vi "Wait Lockin Start.vi"(8 "error in (no error)":errorcluster, 11 "MeasurementSMO in":refnum<class "MeasurementSMO.lvclass">) -> (0 "error out":errorcluster, 3 "MeasurementSMO out":refnum<class "MeasurementSMO.lvclass">)   [LabVIEW 2019, in "MeasurementSMO.lvclass"]
uses:
  MeasurementSMO.lvclass
  14575ef7-ffd8-4de4-94d8-a49df30f0b8f.vi
  <userlib>/LevyLab/Lockin-Multichannel/Instrument.Lockin/Instrument.Lockin.lvclass
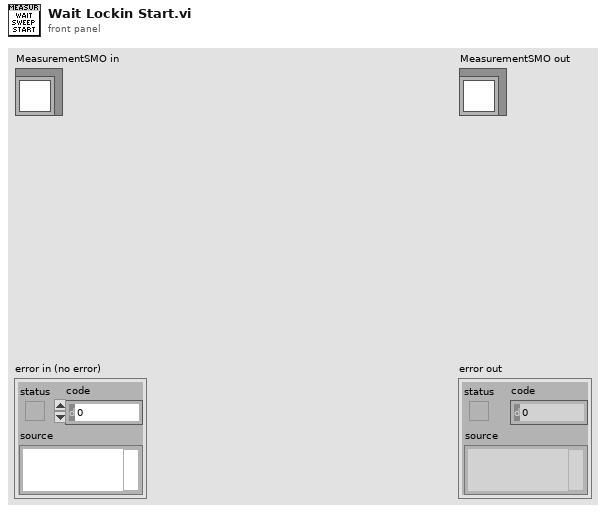
[diagram p1: front panel]
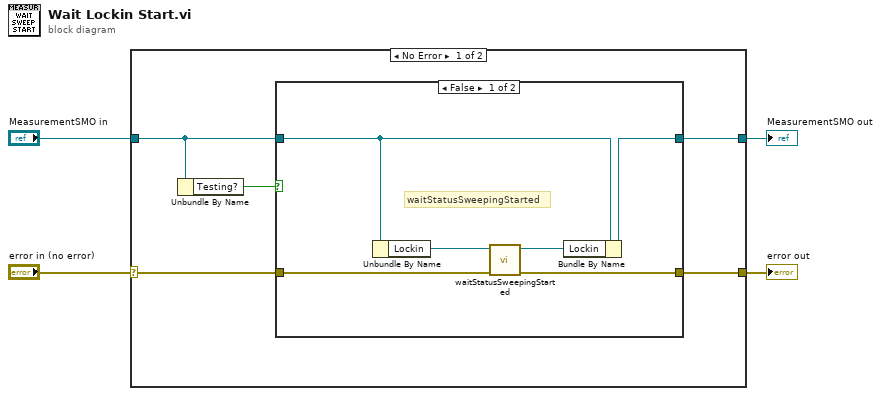
[diagram p0: block diagram]
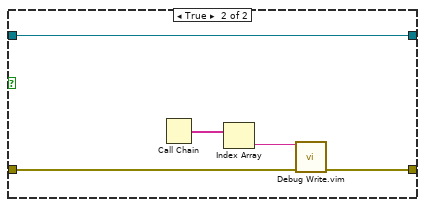
[diagram p2: hidden frame]
diagram:
  n1 = case shown="No Error" "error in (no error)" {
    selector: "error in (no error)" -> [w6 w22]
    tunnel: [w7 w22] -> w3
    tunnel: [w8 w21] -> w1
    tunnel: "MeasurementSMO in" -> [w9 w21]
    frame No Error {
      n2 = Unbundle By Name(w9) -> ("Testing?"=w5:bool)
      n3 = case shown="False" w5 {
        tunnel: w9 -> [w14 w20]
        tunnel: [w15 w20] -> w8
        tunnel: [w10 w19] -> w7
        tunnel: w6 -> [w11 w18]
        frame False {
          # "waitStatusSweepingStarted"
          n4 = Unbundle By Name(w14) -> ("Lockin"=w13:refnum<class "Instrument.Lockin.lvclass">)
          n5 = call <userlib>:"waitStatusSweepingStarted.vi"("error in (no error)"=w11, "Instrument.Lockin in"=w13) -> ("error out"=w10:errorcluster, "Instrument.Lockin out"=w12:refnum<class "Instrument.Lockin.lvclass">)  [unwired: 8 in]
          n6 = Bundle By Name(cluster=w14, "Lockin"=w12) -> (w15:refnum<class "MeasurementSMO.lvclass">)
        }
        frame True {
          n7 = Call Chain() -> (call chain=w16:string[])
          n8 = Index Array(array=w16) -> (element=w17:string)  [unwired: 1 in]
          n9 = call "Debug Write.vim"("error in (no error)"=w18, "value"=w17) -> ("error out"=w19:errorcluster)  [unwired: 9 in]
        }
      }
    }
    frame Error {
    }
  }
  "error out" <- w3
  "MeasurementSMO out" <- w1
